vi "Select Multiple Nodes.vi"(8 "Node to Select":T1={"Node Type"=enum."Path", "ID"=0, "Path Data"={"Path Name"="", "Outcome Name"=""}, "Single Cmd Info"={"Name"="", "CPTM.DataType"=variant, "All Control Values Variant"=[], "icon full"={"image type"=0, "image depth"=0, "image"=[], "mask"=[], "colors"=[], "Rectangle"={"left"=0, "top"=0, "right"=0, "bottom"=0}}, "icon scaled"={"image type"=0, "image depth"=0, "image"=[], "mask"=[], "colors"=[], "Rectangle"={"left"=0, "top"=0, "right"=0, "bottom"=0}}, "Path"=path "", "Subsystem Color"=16777216}, "Child ID"=[], "Parent ID"=0, "Drawing Info"={"X"=0, "Y"=0, "Width"=0, "Height"=0}}, 9 "Selected Nodes":T1[](array[typedef])) -> (0 "New Node":T1, 1 "Selected Nodes New":T1[](array[typedef]))   [LabVIEW 2025]
uses:
  Types/Sequencing Tree Node.ctl
  Types/Single Cmd Info.ctl
  <vilib>/picture/picture.llb/imagedata.ctl
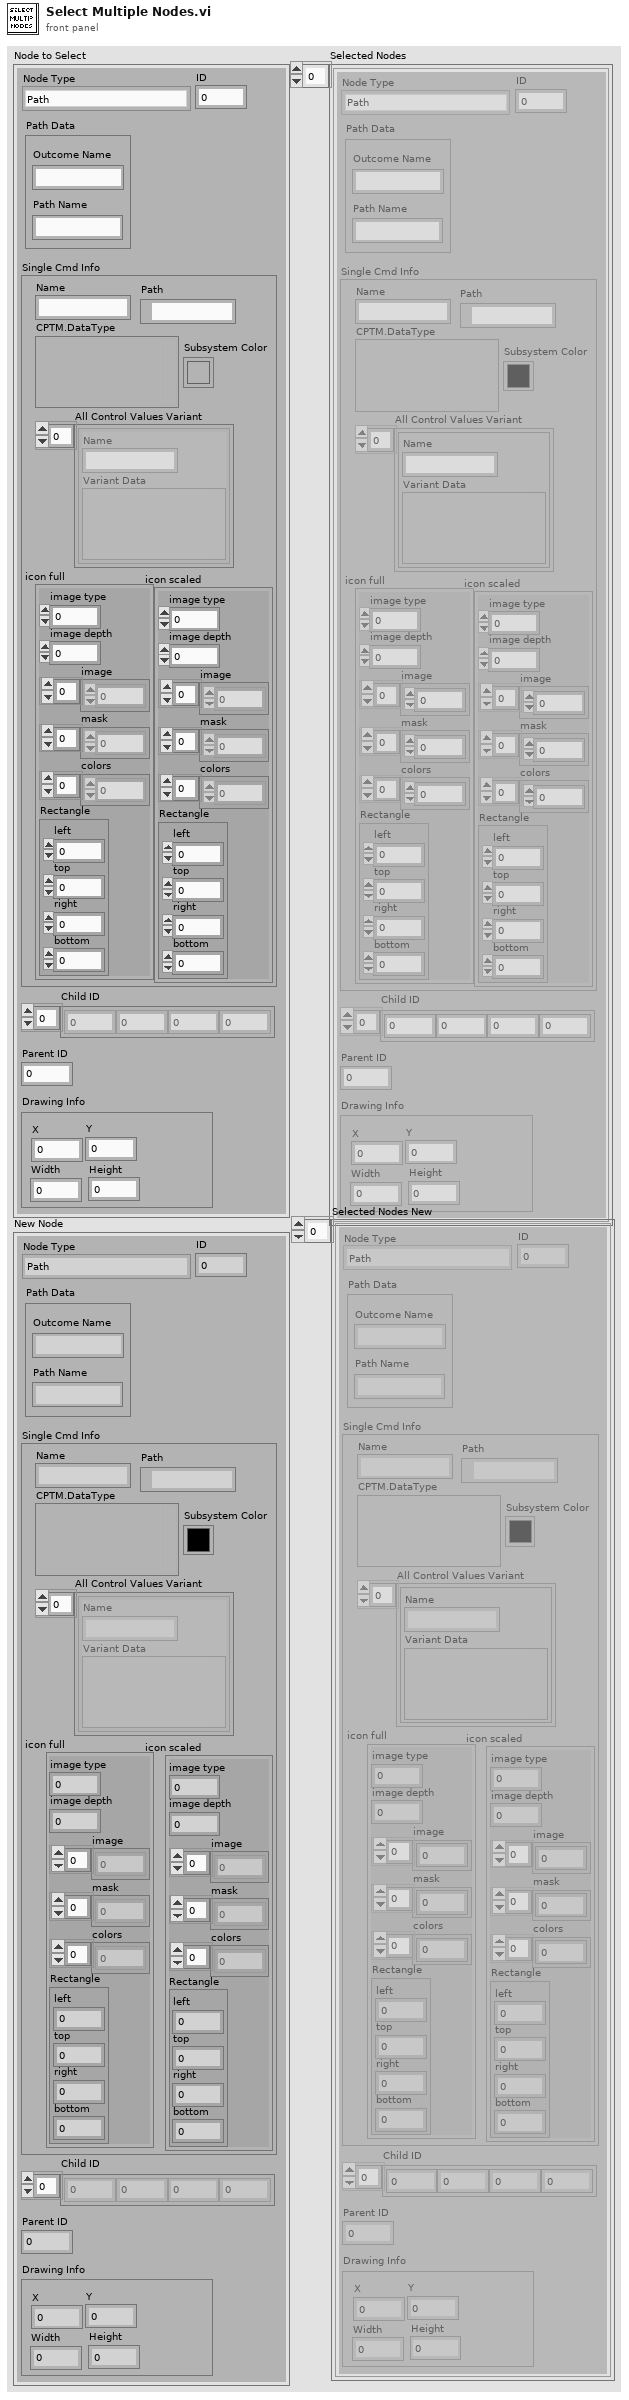
[diagram p1: front panel]
types:
  T1 = typedef "Sequencing Tree Node.ctl" = cluster{"Node Type":enum16{"Path", "Command", "Leaf"}, "ID":i16, "Path Data":cluster{"Path Name":string, "Outcome Name":string}, "Single Cmd Info":T2, "Child ID":i32[], "Parent ID":i32, "Drawing Info":cluster{"X":i32, "Y":i32, "Width":i32, "Height":i32}}
  T2 = typedef "Single Cmd Info.ctl" = cluster{"Name":string, "CPTM.DataType":variant, "All Control Values Variant":cluster{"Name":string, "Variant Data":variant}[], "icon full":T3, "icon scaled":T3, "Path":path, "Subsystem Color":u32}
  T3 = typedef "imagedata.ctl" = cluster{"image type":i32, "image depth":i32, "image":u8[], "mask":u8[], "colors":u32[], "Rectangle":cluster{"left":i16, "top":i16, "right":i16, "bottom":i16}}
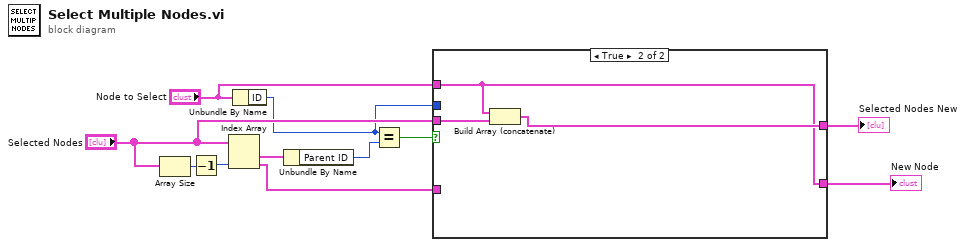
[diagram p0: block diagram]
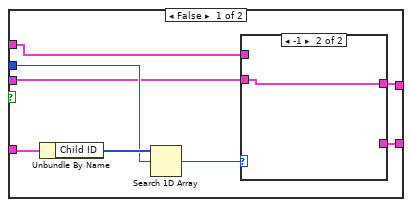
[diagram p2: hidden frame]
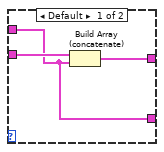
[diagram p3: hidden frame]
diagram:
  n1 = Array Size(array="Selected Nodes") -> (size(s)=w11:i32)
  n2 = Decrement(x=w11) -> (x-1=w10:i32)
  n3 = Index Array(array="Selected Nodes", index #2=w10) -> (element #1=w9:T1, element #2=w4:T1)  [unwired: 1 in]
  n4 = Unbundle By Name("Node to Select") -> ("ID"=w3:i16)
  n5 = Unbundle By Name(w9) -> ("Parent ID"=w8:i32)
  n6 = Equal?(x=w3, y=w8) -> (x = y?=w7:bool)
  n7 = case shown="True" w7 {
    tunnel: "Selected Nodes" -> [w15 w26]
    tunnel: "Node to Select" -> [w14 w24]
    tunnel: w4 -> [w19 _]
    tunnel: w3 -> [w17 _]
    tunnel: [w13 w25] -> w2
    tunnel: [w12 w24] -> w1
    frame False {
      n8 = Unbundle By Name(w19) -> ("Child ID"=w18:i32[])
      n9 = Search 1D Array(1D array=w18, element=w17) -> (index of element=w16:i32)  [unwired: 1 in]
      n10 = case shown="-1" w16 {
        tunnel: w15 -> [w22 w23]
        tunnel: w14 -> [w20 _]
        tunnel: [w21 w23] -> w13
        tunnel: [w20 _] -> w12
        frame Default {
          n11 = Build Array (concatenate)(w22, w20) -> (w21:T1[])
        }
        frame -1 {
        }
      }
    }
    frame True {
      n12 = Build Array (concatenate)(w24, w26) -> (w25:T1[])
    }
  }
  "Selected Nodes New" <- w2
  "New Node" <- w1
